vi "Write Image Data to Gif File.vi"(8 "error in (no error)":errorcluster caption="错误输入（无错误）", 10 "image data":T1 caption="图像数据", 11 "path to GIF file":path caption="GIF文件路径") -> (0 "error out":errorcluster caption="错误输出", 3 "path":path caption="路径")   [LabVIEW 2011, in "Gif Image.lvclass"]
uses:
  Gif Image.lvclass
  <vilib>/picture/picture.llb/imagedata.ctl
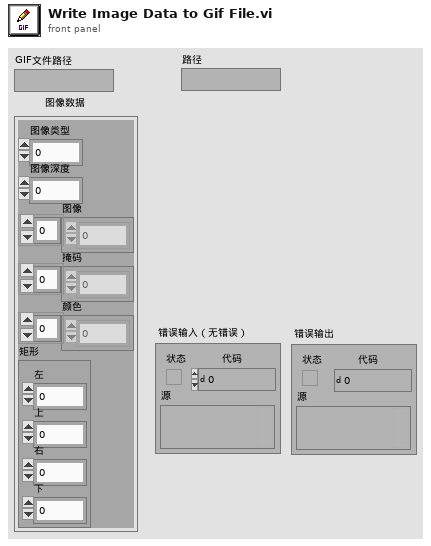
[diagram p1: front panel]
types:
  T1 = typedef "imagedata.ctl" = cluster{"image type":i32, "image depth":i32, "image":u8[], "mask":u8[], "colors":u32[], "Rectangle":cluster{"left":i16, "top":i16, "right":i16, "bottom":i16}}
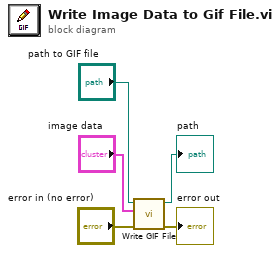
[diagram p0: block diagram]
diagram:
  n1 = call <vilib>:"Write GIF File.vi"("error in (no error)"="error in (no error)", "image data"="image data", "path to GIF file"="path to GIF file") -> ("error out"=→"error out":errorcluster, "path"=→"path":path)  [unwired: 7 in]
